vi "Lab Panel V5.25.vi"() -> ()   [LabVIEW 2017] (continued)
                    n2903 = Unbundle(w5372) -> ("CYCLE"=w5336:dbl, "MINS"=w5335:dbl, "STATUS"=w5332:string)
                    n2904 = Unbundle(w5371) -> ("CYCLE"=w5331:dbl, "MINS"=w5330:dbl, "STATUS"=w5327:string)
                    n2905 = Unbundle(w5370) -> ("CYCLE"=w5326:dbl, "MINS"=w5325:dbl, "STATUS"=w5322:string)
                    n2906 = Unbundle(w5369) -> ("CYCLE"=w5368:dbl, "MINS"=w5367:dbl, "STATUS"=w5319:string)
                    n2907 = Number To Decimal String(number=w5354) -> (decimal integer string=w5356:string)  [unwired: 1 in]
                    n2908 = Number To Decimal String(number=w5351) -> (decimal integer string=w5349:string)  [unwired: 1 in]
                    n2909 = Number To Decimal String(number=w5346) -> (decimal integer string=w5344:string)  [unwired: 1 in]
                    n2910 = Number To Decimal String(number=w5361) -> (decimal integer string=w5359:string)  [unwired: 1 in]
                    n2911 = Number To Decimal String(number=w5341) -> (decimal integer string=w5339:string)  [unwired: 1 in]
                    n2912 = Number To Decimal String(number=w5366) -> (decimal integer string=w5364:string)  [unwired: 1 in]
                    n2913 = Number To Decimal String(number=w5368) -> (decimal integer string=w5321:string)  [unwired: 1 in]
                    n2914 = Number To Decimal String(number=w5336) -> (decimal integer string=w5334:string)  [unwired: 1 in]
                    n2915 = Number To Decimal String(number=w5331) -> (decimal integer string=w5329:string)  [unwired: 1 in]
                    n2916 = Number To Decimal String(number=w5326) -> (decimal integer string=w5324:string)  [unwired: 1 in]
                    n2917 = Number To Fractional String(number=w5353, precision (6)=w5298) -> (F-format string=w5355:string)  [unwired: 2 in]
                    n2918 = Number To Fractional String(number=w5340, precision (6)=w5298) -> (F-format string=w5338:string)  [unwired: 2 in]
                    n2919 = Number To Fractional String(number=w5350, precision (6)=w5298) -> (F-format string=w5348:string)  [unwired: 2 in]
                    n2920 = Number To Fractional String(number=w5345, precision (6)=w5298) -> (F-format string=w5343:string)  [unwired: 2 in]
                    n2921 = Number To Fractional String(number=w5330, precision (6)=w5298) -> (F-format string=w5328:string)  [unwired: 2 in]
                    n2922 = Number To Fractional String(number=w5335, precision (6)=w5298) -> (F-format string=w5333:string)  [unwired: 2 in]
                    n2923 = Number To Fractional String(number=w5360, precision (6)=w5298) -> (F-format string=w5358:string)  [unwired: 2 in]
                    n2924 = Number To Fractional String(number=w5325, precision (6)=w5298) -> (F-format string=w5323:string)  [unwired: 2 in]
                    n2925 = Number To Fractional String(number=w5365, precision (6)=w5298) -> (F-format string=w5363:string)  [unwired: 2 in]
                    n2926 = Number To Fractional String(number=w5367, precision (6)=w5298) -> (F-format string=w5320:string)  [unwired: 2 in]
                    n2927 = Concatenate Strings(w5297, w5339, w5297, w5338, w5297, w5337) -> (w5313:string)
                    n2928 = Concatenate Strings(w5297, w5334, w5297, w5333, w5297, w5332) -> (w5312:string)
                    n2929 = Concatenate Strings(w5297, w5329, w5297, w5328, w5297, w5327) -> (w5311:string)
                    n2930 = Concatenate Strings(w5297, w5324, w5297, w5323, w5297, w5322) -> (w5310:string)
                    n2931 = Concatenate Strings(w5297, w5321, w5297, w5320, w5297, w5319) -> (w5309:string)
                    n2932 = Concatenate Strings(w5297, w5364, w5297, w5363, w5297, w5362) -> (w5318:string)
                    n2933 = Concatenate Strings(w5297, w5344, w5297, w5343, w5297, w5342) -> (w5314:string)
                    n2934 = Concatenate Strings(w5297, w5359, w5297, w5358, w5297, w5357) -> (w5317:string)
                    n2935 = Concatenate Strings(w5297, w5356, w5297, w5355, w5297, w5352) -> (w5316:string)
                    n2936 = Concatenate Strings(w5297, w5349, w5297, w5348, w5297, w5347) -> (w5315:string)
                    n2937 = Concatenate Strings("]", "\r") -> (w5294:string)
                    n2938 = Concatenate Strings(w5289, w5314, w5294) -> (w5304:string)
                    n2939 = Concatenate Strings(w5291, w5316, w5294) -> (w5306:string)
                    n2940 = Concatenate Strings(w5290, w5315, w5294) -> (w5305:string)
                    n2941 = Concatenate Strings(w5286, w5311, w5294) -> (w5301:string)
                    n2942 = Concatenate Strings(w5287, w5310, w5294) -> (w5302:string)
                    n2943 = Concatenate Strings(w5285, w5312, w5294) -> (w5300:string)
                    n2944 = Concatenate Strings(w5284, w5313, w5294) -> (w5299:string)
                    n2945 = Concatenate Strings(w5288, w5309, w5294) -> (w5303:string)
                    n2946 = Concatenate Strings(w5292, w5317, w5294) -> (w5307:string)
                    n2947 = Concatenate Strings(w5293, w5318, w5294) -> (w5308:string)
                    n2948 = Concatenate Strings(w5308, w5307, w5306, w5305, w5304, w5299, w5300, w5301, w5302, w5303) -> (w5277:string)
                    n2949 = Concatenate Strings("[PANEL/", "DESC/", "CYCLES/", "MINS/", "STATUS]", "\r", w5277) -> (w5276:string)
                    "MAIL REPORT" <- w5276
                    n2950 = global write "Global display 3.vi" "log all"(w5276) -> ()
                  }
                  frame #2 {
                    w5407 = "END"
                    n2951 = local read "mail control"() -> (w5408:string)
                    n2952 = case shown="False" w5403 {
                      tunnel: w5408 -> [w5432 _]
                      tunnel: w5407 -> [w5431 _]
                      tunnel: [w5430 FALSE] -> w5393
                      frame False {
                        n2953 = Equal?(x=w5432, y=w5431) -> (x = y?=w5430:bool)
                      }
                      frame True {
                      }
                    }
                    n2954 = case shown="False" w5409 {
                      tunnel: w5408 -> [w5448 _]
                      tunnel: w5407 -> [w5447 _]
                      tunnel: [w5446 FALSE] -> w5397
                      frame False {
                        n2955 = Equal?(x=w5448, y=w5447) -> (x = y?=w5446:bool)
                      }
                      frame True {
                      }
                    }
                    n2956 = case shown="False" w5406 {
                      tunnel: w5408 -> [w5444 _]
                      tunnel: w5407 -> [w5443 _]
                      tunnel: [w5442 FALSE] -> w5396
                      frame False {
                        n2957 = Equal?(x=w5444, y=w5443) -> (x = y?=w5442:bool)
                      }
                      frame True {
                      }
                    }
                    n2958 = case shown="False" w5404 {
                      tunnel: w5408 -> [w5436 _]
                      tunnel: w5407 -> [w5435 _]
                      tunnel: [w5434 FALSE] -> w5394
                      frame False {
                        n2959 = Equal?(x=w5436, y=w5435) -> (x = y?=w5434:bool)
                      }
                      frame True {
                      }
                    }
                    n2960 = case shown="False" w5405 {
                      tunnel: w5408 -> [w5440 _]
                      tunnel: w5407 -> [w5439 _]
                      tunnel: [w5438 FALSE] -> w5395
                      frame False {
                        n2961 = Equal?(x=w5440, y=w5439) -> (x = y?=w5438:bool)
                      }
                      frame True {
                      }
                    }
                    n2962 = Or(x=w5395, y=w5394) -> (x .or. y?=w5386:bool)
                    n2963 = Or(x=w5397, y=w5396) -> (x .or. y?=w5387:bool)
                    n2964 = Or(x=w5387, y=w5386) -> (x .or. y?=w5382:bool)
                    n2965 = case shown="False" w5399 {
                      tunnel: w5408 -> [w5416 _]
                      tunnel: w5407 -> [w5415 _]
                      tunnel: [w5414 FALSE] -> w5388
                      frame False {
                        n2966 = Equal?(x=w5416, y=w5415) -> (x = y?=w5414:bool)
                      }
                      frame True {
                      }
                    }
                    n2967 = case shown="False" w5398 {
                      tunnel: w5408 -> [w5412 _]
                      tunnel: w5407 -> [w5411 _]
                      tunnel: [w5410 FALSE] -> w5392
                      frame False {
                        n2968 = Equal?(x=w5412, y=w5411) -> (x = y?=w5410:bool)
                      }
                      frame True {
                      }
                    }
                    n2969 = case shown="False" w5400 {
                      tunnel: w5408 -> [w5420 _]
                      tunnel: w5407 -> [w5419 _]
                      tunnel: [w5418 FALSE] -> w5389
                      frame False {
                        n2970 = Equal?(x=w5420, y=w5419) -> (x = y?=w5418:bool)
                      }
                      frame True {
                      }
                    }
                    n2971 = case shown="False" w5402 {
                      tunnel: w5408 -> [w5428 _]
                      tunnel: w5407 -> [w5427 _]
                      tunnel: [w5426 FALSE] -> w5391
                      frame False {
                        n2972 = Equal?(x=w5428, y=w5427) -> (x = y?=w5426:bool)
                      }
                      frame True {
                      }
                    }
                    n2973 = case shown="False" w5401 {
                      tunnel: w5408 -> [w5424 _]
                      tunnel: w5407 -> [w5423 _]
                      tunnel: [w5422 FALSE] -> w5390
                      frame False {
                        n2974 = Equal?(x=w5424, y=w5423) -> (x = y?=w5422:bool)
                      }
                      frame True {
                      }
                    }
                    n2975 = Or(x=w5391, y=w5390) -> (x .or. y?=w5385:bool)
                    n2976 = Or(x=w5389, y=w5388) -> (x .or. y?=w5384:bool)
                    n2977 = Or(x=w5392, y=w5393) -> (x .or. y?=w5380:bool)
                    n2978 = Or(x=w5385, y=w5384) -> (x .or. y?=w5383:bool)
                    n2979 = Or(x=w5382, y=w5383) -> (x .or. y?=w5381:bool)
                    n2980 = Or(x=w5381, y=w5380) -> (x .or. y?=w5379:bool)
                  }
                  frame #3 {
                    n2981 = local read "on loops"() -> (w5462:dbl)
                    n2982 = local read "jig cycle"() -> (w5459:dbl)
                    n2983 = local read "Send Mail Now"() -> (w5453:bool)
                    n2984 = Add(x=w5462, y=3.0) -> (x+y=w5460:dbl)
                    n2985 = Equal?(x=w5459, y=w5460) -> (x = y?=w5454:bool)
                    n2986 = And(x=w5454, y=w5453) -> (x .and. y?=w5452:bool)
                    n2987 = And(x=w5458, y=w5454) -> (x .and. y?=w5457:bool)
                    n2988 = And(x=w5457, y=w5456) -> (x .and. y?=w5455:bool)
                    n2989 = Or(x=w5455, y=w5452) -> (x .or. y?=w5451:bool)
                    n2990 = case shown="True" w5451 {
                      tunnel: w5467 -> [_ w5473]
                      tunnel: w5466 -> [_ w5472]
                      tunnel: "Lab Panel Test Status" -> [_ w5471]
                      tunnel: w5464 -> [_ w5470]
                      tunnel: w5463 -> [_ w5469]
                      tunnel: w5450 -> [_ w5468]
                      frame False {
                      }
                      frame True {
                        n2991 = stacked-sequence {
                          tunnel: w5473 -> [w5481 _]
                          tunnel: w5472 -> [w5480 _]
                          tunnel: w5471 -> [w5479 _]
                          tunnel: w5470 -> [w5478 _]
                          tunnel: w5469 -> [w5477 _]
                          tunnel: w5468 -> [w5476 _]
                          frame #0 {
                            n2992 = call "Lab Send Mail Test.vi"("TO:"=w5481, "subject"=w5479, "from"=w5477, "out going server"=w5478, "message"=w5480) -> ("error out"=w5475:errorcluster)  [unwired: 10 in]
                            n2993 = Bundle(cluster=w5476, "mail error"=w5475) -> (w5474:T7)  [unwired: 6 in]
                            n2994 = local write "MAIL SETTINGS"(w5474) -> ()
                          }
                          frame #1 {
                            n2995 = local write "mail control"("") -> ()
                            n2996 = local write "Send Mail Now"(FALSE) -> ()
                          }
                        }
                      }
                    }
                  }
                }
              }
            }
          }
          frame #19 {
            # "save jig cycle values once all run switches are off"
            n2997 = stacked-sequence {
              tunnel: w5493 -> [_ w5522]
              tunnel: w5492 -> [_ w5521]
              tunnel: w5491 -> [_ w5520]
              tunnel: w5490 -> [_ w5519]
              tunnel: w5489 -> [_ w5518]
              tunnel: w5488 -> [_ w5517]
              tunnel: w5487 -> [_ w5516]
              tunnel: w5486 -> [_ w5515]
              tunnel: w5485 -> [_ w5514]
              tunnel: w5484 -> [_ w5513]
              frame #0 {
              }
              frame #1 {
                n2998 = Not(x=w5513) -> (.not. x?=w5496:bool)
                n2999 = Not(x=w5521) -> (.not. x?=w5511:bool)
                n3000 = Not(x=w5518) -> (.not. x?=w5506:bool)
                n3001 = Not(x=w5516) -> (.not. x?=w5502:bool)
                n3002 = Not(x=w5514) -> (.not. x?=w5498:bool)
                n3003 = Not(x=w5522) -> (.not. x?=w5512:bool)
                n3004 = Not(x=w5520) -> (.not. x?=w5510:bool)
                n3005 = Not(x=w5517) -> (.not. x?=w5504:bool)
                n3006 = Not(x=w5519) -> (.not. x?=w5508:bool)
                n3007 = Not(x=w5515) -> (.not. x?=w5500:bool)
                n3008 = local read "Save JC"() -> (w5524:bool)
                n3009 = And(x=w5512, y=w5511) -> (x .and. y?=w5509:bool)
                n3010 = And(x=w5509, y=w5510) -> (x .and. y?=w5507:bool)
                n3011 = And(x=w5507, y=w5508) -> (x .and. y?=w5505:bool)
                n3012 = And(x=w5505, y=w5506) -> (x .and. y?=w5503:bool)
                n3013 = And(x=w5503, y=w5504) -> (x .and. y?=w5501:bool)
                n3014 = And(x=w5501, y=w5502) -> (x .and. y?=w5499:bool)
                n3015 = And(x=w5499, y=w5500) -> (x .and. y?=w5497:bool)
                n3016 = And(x=w5497, y=w5498) -> (x .and. y?=w5495:bool)
                n3017 = And(x=w5495, y=w5496) -> (x .and. y?=w5494:bool)
                n3018 = And(x=w5494, y=w5524) -> (x .and. y?=w5523:bool)
                n3019 = case shown="True" w5523 {
                  tunnel: w5494 -> [w5525 _]
                  frame False {
                    n3020 = case shown="False" w5525 {
                      frame False {
                        n3021 = local write "Save JC"(TRUE) -> ()
                      }
                      frame True {
                      }
                    }
                  }
                  frame True {
                    n3022 = stacked-sequence {
                      frame #0 {
                        n3023 = String To Path(string="c:\\crabtree\\Jig Cycles\\") -> (path=w5537:path)
                        n3024 = Build Path(base path=w5537, name or relative path="jigcycles.bin") -> (appended path=w5535:path)
                        n3025 = Create Folder(path (use dialog)=w5537) -> (error out=w5539:errorcluster)  [unwired: 2 in, 2 out]
                        n3026 = local read "JIG RELAY CYCLES"() -> (w5529:T8)
                        n3027 = call <vilib>:"Clear Errors.vi"("error in (no error)"=w5539) -> ()  [unwired: 5 in, 2 out]
                        n3028 = local write "Save JC"(FALSE) -> ()
                        n3029 = Open/Create/Replace File(file path (use dialog)=w5535, operation (0:open)=T17."replace or create") -> (refnum out=w5533:refnum<file>, error out=w5534:errorcluster)  [unwired: 4 in, 1 out]
                        n3030 = Write to Binary File(file (use dialog)=w5533, data=w5529, error in=w5534) -> (refnum out=w5532:refnum<file>, error out=w5531:errorcluster)  [unwired: 3 in, 1 out]
                        n3031 = Close File(refnum=w5532, error in=w5531) -> (error out=w5530:errorcluster)  [unwired: 1 out]
                        n3032 = local write "data file error"(w5530) -> ()
                      }
                      frame #1 {
                        n3033 = local read "JIG RELAY CYCLES"() -> (w5562:T8)
                        n3034 = Unbundle By Name(w5562) -> ("LAB01-1"=w5557:dbl, "LAB01-2"=w5556:dbl, "LAB02-1"=w5554:dbl, "LAB02-2"=w5553:dbl, "LAB03-1"=w5551:dbl, "LAB03-2"=w5548:dbl, "LAB04-1"=w5547:dbl, "LAB04-2"=w5545:dbl, "LAB05-1"=w5543:dbl, "LAB05-2"=w5541:dbl)
                        n3035 = stacked-sequence {
                          tunnel: w5557 -> [w5565 _ _ _ _ _ _ _ _ _]
                          tunnel: 1000000 -> [w5568 w5578 w5588 w5598 w5608 w5618 w5628 w5638 w5648 w5658]
                          tunnel: [w5566 _ _ _ _ _ _ _ _ _] -> w5560
                          tunnel: "TEST STATION HAS REACHED 1 MILLION CYCLES, REPLACE  CONTROL RELAYS" -> [w5564 w5576 w5586 w5596 w5606 w5616 w5626 w5636 w5646 w5656]
                          tunnel: [_ w5575 _ _ _ _ _ _ _ _] -> w5558
                          tunnel: w5556 -> [_ w5574 _ _ _ _ _ _ _ _]
                          tunnel: [_ _ w5585 _ _ _ _ _ _ _] -> w5555
                          tunnel: w5554 -> [_ _ w5584 _ _ _ _ _ _ _]
                          tunnel: w5553 -> [_ _ _ w5595 _ _ _ _ _ _]
                          tunnel: [_ _ _ w5594 _ _ _ _ _ _] -> w5552
                          tunnel: w5551 -> [_ _ _ _ w5605 _ _ _ _ _]
                          tunnel: [_ _ _ _ w5604 _ _ _ _ _] -> w5550
                          tunnel: [_ _ _ _ _ w5615 _ _ _ _] -> w5549
                          tunnel: w5548 -> [_ _ _ _ _ w5614 _ _ _ _]
                          tunnel: w5547 -> [_ _ _ _ _ _ w5625 _ _ _]
                          tunnel: [_ _ _ _ _ _ w5624 _ _ _] -> w5546
                          tunnel: w5545 -> [_ _ _ _ _ _ _ w5635 _ _]
                          tunnel: [_ _ _ _ _ _ _ w5634 _ _] -> w5544
                          tunnel: w5543 -> [_ _ _ _ _ _ _ _ w5645 _]
                          tunnel: [_ _ _ _ _ _ _ _ w5644 _] -> w5542
                          tunnel: w5541 -> [_ _ _ _ _ _ _ _ _ w5655]
                          tunnel: [_ _ _ _ _ _ _ _ _ w5654] -> w5540
                          frame #0 {
                            n3036 = Greater?(x=w5565, y=w5568) -> (0:w5567:bool)
                            n3037 = case shown="True" w5567 {
                              tunnel: [w5569 0] -> w5566
                              tunnel: w5565 -> [w5569 _]
                              tunnel: w5564 -> [_ w5570]
                              frame False {
                              }
                              frame True {
                                n3038 = Concatenate Strings("LA01-1 ", w5570) -> (w5573:string)
                                n3039 = One Button Dialog(message=w5573) -> ()  [unwired: 1 in, 1 out]
                              }
                            }
                          }
                          frame #1 {
                            n3040 = Greater?(x=w5574, y=w5578) -> (0:w5577:bool)
                            n3041 = case shown="True" w5577 {
                              tunnel: [w5579 0] -> w5575
                              tunnel: w5574 -> [w5579 _]
                              tunnel: w5576 -> [_ w5580]
                              frame False {
                              }
                              frame True {
                                n3042 = Concatenate Strings("LA01-2 ", w5580) -> (w5583:string)
                                n3043 = One Button Dialog(message=w5583) -> ()  [unwired: 1 in, 1 out]
                              }
                            }
                          }
                          frame #2 {
                            n3044 = Greater?(x=w5584, y=w5588) -> (0:w5587:bool)
                            n3045 = case shown="True" w5587 {
                              tunnel: [w5589 0] -> w5585
                              tunnel: w5584 -> [w5589 _]
                              tunnel: w5586 -> [_ w5590]
                              frame False {
                              }
                              frame True {
                                n3046 = Concatenate Strings("LA02-1 ", w5590) -> (w5593:string)
                                n3047 = One Button Dialog(message=w5593) -> ()  [unwired: 1 in, 1 out]
                              }
                            }
                          }
                          frame #3 {
                            n3048 = Greater?(x=w5595, y=w5598) -> (0:w5597:bool)
                            n3049 = case shown="True" w5597 {
                              tunnel: [w5599 0] -> w5594
                              tunnel: w5595 -> [w5599 _]
                              tunnel: w5596 -> [_ w5600]
                              frame False {
                              }
                              frame True {
                                n3050 = Concatenate Strings("LA02-2 ", w5600) -> (w5603:string)
                                n3051 = One Button Dialog(message=w5603) -> ()  [unwired: 1 in, 1 out]
                              }
                            }
                          }
                          frame #4 {
                            n3052 = Greater?(x=w5605, y=w5608) -> (0:w5607:bool)
                            n3053 = case shown="True" w5607 {
                              tunnel: [w5609 0] -> w5604
                              tunnel: w5605 -> [w5609 _]
                              tunnel: w5606 -> [_ w5610]
                              frame False {
                              }
                              frame True {
                                n3054 = Concatenate Strings("LA03-1 ", w5610) -> (w5613:string)
                                n3055 = One Button Dialog(message=w5613) -> ()  [unwired: 1 in, 1 out]
                              }
                            }
                          }
                          frame #5 {
                            n3056 = Greater?(x=w5614, y=w5618) -> (0:w5617:bool)
                            n3057 = case shown="True" w5617 {
                              tunnel: [w5619 0] -> w5615
                              tunnel: w5614 -> [w5619 _]
                              tunnel: w5616 -> [_ w5620]
                              frame False {
                              }
                              frame True {
                                n3058 = Concatenate Strings("LA03-2 ", w5620) -> (w5623:string)
                                n3059 = One Button Dialog(message=w5623) -> ()  [unwired: 1 in, 1 out]
                              }
                            }
                          }
                          frame #6 {
                            n3060 = Greater?(x=w5625, y=w5628) -> (0:w5627:bool)
                            n3061 = case shown="True" w5627 {
                              tunnel: [w5629 0] -> w5624
                              tunnel: w5625 -> [w5629 _]
                              tunnel: w5626 -> [_ w5630]
                              frame False {
                              }
                              frame True {
                                n3062 = Concatenate Strings("LA04-1 ", w5630) -> (w5633:string)
                                n3063 = One Button Dialog(message=w5633) -> ()  [unwired: 1 in, 1 out]
                              }
                            }
                          }
                          frame #7 {
                            n3064 = Greater?(x=w5635, y=w5638) -> (0:w5637:bool)
                            n3065 = case shown="True" w5637 {
                              tunnel: [w5639 0] -> w5634
                              tunnel: w5635 -> [w5639 _]
                              tunnel: w5636 -> [_ w5640]
                              frame False {
                              }
                              frame True {
                                n3066 = Concatenate Strings("LA04-2 ", w5640) -> (w5643:string)
                                n3067 = One Button Dialog(message=w5643) -> ()  [unwired: 1 in, 1 out]
                              }
                            }
                          }
                          frame #8 {
                            n3068 = Greater?(x=w5645, y=w5648) -> (0:w5647:bool)
                            n3069 = case shown="True" w5647 {
                              tunnel: [w5649 0] -> w5644
                              tunnel: w5645 -> [w5649 _]
                              tunnel: w5646 -> [_ w5650]
                              frame False {
                              }
                              frame True {
                                n3070 = Concatenate Strings("LA05-1 ", w5650) -> (w5653:string)
                                n3071 = One Button Dialog(message=w5653) -> ()  [unwired: 1 in, 1 out]
                              }
                            }
                          }
                          frame #9 {
                            n3072 = Greater?(x=w5655, y=w5658) -> (0:w5657:bool)
                            n3073 = case shown="True" w5657 {
                              tunnel: [w5659 0] -> w5654
                              tunnel: w5655 -> [w5659 _]
                              tunnel: w5656 -> [_ w5660]
                              frame False {
                              }
                              frame True {
                                n3074 = Concatenate Strings("LA05-2 ", w5660) -> (w5663:string)
                                n3075 = One Button Dialog(message=w5663) -> ()  [unwired: 1 in, 1 out]
                              }
                            }
                          }
                        }
                        n3076 = Bundle By Name(cluster=w5562, "LAB01-1"=w5560, "LAB01-2"=w5558, "LAB02-1"=w5555, "LAB02-2"=w5552, "LAB03-1"=w5550, "LAB03-2"=w5549, "LAB04-1"=w5546, "LAB04-2"=w5544, "LAB05-1"=w5542, "LAB05-2"=w5540) -> (w5561:T8)
                        n3077 = local write "JIG RELAY CYCLES"(w5561) -> ()
                      }
                    }
                  }
                }
              }
            }
          }
          frame #20 {
            # "get temperature values"
            n3078 = local read "Simulate"() -> (w5676:bool)
            n3079 = local read "Temp Test Cal"() -> (w5673:dbl)
            n3080 = stacked-sequence {
              seq-local: [w5678 _] -> [_ w5723]
              tunnel: w5676 -> [_ w5736]
              tunnel: T14 {"1  (A) cal"=1.0, "1 (V) cal"=1.0, "1 (PF) cal"=1.0, "1 (TL) cal"=1.0, "1 (TN) cal"=1.0, "2 (A) cal"=1.0, "2 (V) cal"=1.0, "2 (PF) cal"=1.0, "2 (TL) cal"=1.0, "2 (TN) cal"=1.0} ("CAL LAB01") -> [_ w5735]
              tunnel: w5674 -> [_ w5734]
              tunnel: w5673 -> [_ w5733]
              tunnel: w5672 -> [_ w5732]
              tunnel: w5671 -> [_ w5731]
              tunnel: w5670 -> [_ w5730]
              tunnel: w5669 -> [_ w5729]
              tunnel: w5668 -> [_ w5728]
              tunnel: w5667 -> [_ w5727]
              tunnel: w5666 -> [_ w5726]
              tunnel: w5665 -> [_ w5725]
              tunnel: w5664 -> [_ w5724]
              frame #0 {
                # "only get temperature from initial valid temperature circuits"
                n3081 = local read "Select COM port"() -> (w5686:refnum<visa-resource-name>)
                "COM port" <- w5686
                n3082 = global write "Global 1.vi" "COM port"(w5686) -> ()
                n3083 = global write "Global 1.vi" "tmp dly lps"("Temp Delay Lps") -> ()
                n3084 = local read "Temp read loop"() -> (w5683:dbl)
                n3085 = global write "Global 1.vi" "dly value"("Temp Value") -> ()
                n3086 = local read "jig cycle"() -> (w5687:dbl)
                n3087 = local read "on loops"() -> (w5689:dbl)
                n3088 = Equal?(x=w5683, y=1) -> (x = y?=w5680:bool)
                n3089 = Add(x=w5689, y=3) -> (x+y=w5690:dbl)
                n3090 = Equal?(x=w5687, y=w5690) -> (x = y?=w5681:bool)
                n3091 = And(x=w5681, y=w5680) -> (x .and. y?=w5679:bool)
                n3092 = Or(x=w5679, y="Read Temp") -> (x .or. y?=w5678:bool)
                n3093 = case shown="True" w5678 {
                  frame False {
                  }
                  frame True {
                    n3094 = local read "Simulate"() -> (w5692:bool)
                    n3095 = local write "TEMP"(TRUE) -> ()
                    n3096 = local write "Read Temp"(FALSE) -> ()
                    n3097 = stacked-sequence {
                      tunnel: 1.0 -> [_ _ _ _ w5722]
                      tunnel: w5692 -> [_ _ _ _ w5721]
                      frame #0 {
                        # "only switch relay on to reset temp circuits if busy testing"
                        n3098 = disable-structure shown="Disabled" {
                          frame Disabled {
                            n3099 = local read "Any Test Running"() -> ()  [unwired: 1 out]
                          }
                          frame Enabled {
                          }
                        }
                        n3100 = local read "USB OUT 0"() -> (w5696:bool[])
                        n3101 = local read "USB OUT 2"() -> (w5698:bool[])
                        n3102 = local read "USB OUT 1"() -> (w5697:bool[])
                        n3103 = Insert Into Array(array=w5698, index=7, new element=TRUE) -> (w5699:bool[])
                        n3104 = call "sub vi - Drive Relays All v6.vi"("Array #2"=w5699, "Array #1"=w5697, "Array #0"=w5696) -> ()  [unwired: 8 in, 1 out]
                      }
                      frame #1 {
                        # "time delay"
                        n3105 = Wait (ms)(milliseconds to wait=500) -> ()  [unwired: 1 out]
                      }
                      frame #2 {
                        # "switch relay off"
                        n3106 = local read "USB OUT 0"() -> (w5702:bool[])
                        n3107 = local read "USB OUT 2"() -> (w5704:bool[])
                        n3108 = local read "USB OUT 1"() -> (w5703:bool[])
                        n3109 = Insert Into Array(array=w5704, index=7, new element=FALSE) -> (w5705:bool[])
                        n3110 = call "sub vi - Drive Relays All v6.vi"("Array #2"=w5705, "Array #1"=w5703, "Array #0"=w5702) -> ()  [unwired: 8 in, 1 out]
                      }
                      frame #3 {
                        # "time delay"
                        n3111 = Wait (ms)(milliseconds to wait=200) -> ()  [unwired: 1 out]
                      }
                      frame #4 {
                        # "read all valid temp circuits"
                        n3112 = local read "LAB01-TP"() -> (w5714:bool)
                        n3113 = local read "LAB03-TP"() -> (w5712:bool)
                        n3114 = local read "LAB02-TP"() -> (w5713:bool)
                        n3115 = local read "LAB04-TP"() -> (w5711:bool)
                        n3116 = local read "LAB05-TP"() -> (w5715:bool)
                        n3117 = call "sub vi - GET ALL TEMP v7.vi"("LA01-EN"=w5714, "simulate"=w5721, "LA02-EN"=w5713, "LA03-EN"=w5712, "LA04-EN"=w5711, "LA05-EN"=w5715, "Gen Cal Value"=w5722) -> ("LOOP TIME"=→"Read Time":dbl, "LA01 TEMP"=w5720:T25, "LA02 TEMP"=w5719:T25, "LA03 TEMP"=w5718:T25, "LA04 TEMP"=w5717:T25, "error"=→"Error Temp":bool, "LA05 TEMP"=w5716:T25)  [unwired: 1 in, 1 out]
                        n3118 = local write "LAB01 TEMP"(w5720) -> ()
                        n3119 = local write "LAB02 TEMP"(w5719) -> ()
                        n3120 = local write "LAB03 TEMP"(w5718) -> ()
                        n3121 = local write "LAB04 TEMP"(w5717) -> ()
                        n3122 = local write "LAB05 TEMP"(w5716) -> ()
                      }
                    }
                  }
                }
              }
              frame #1 {
                n3123 = case shown="True" w5723 {
                  tunnel: w5736 -> [_ w5749]
                  tunnel: w5735 -> [_ w5748]
                  tunnel: w5734 -> [_ w5747]
                  tunnel: w5733 -> [_ w5746]
                  tunnel: w5732 -> [_ w5745]
                  tunnel: w5731 -> [_ w5744]
                  tunnel: w5730 -> [_ w5743]
                  tunnel: w5729 -> [_ w5742]
                  tunnel: w5728 -> [_ w5741]
                  tunnel: w5727 -> [_ w5740]
                  tunnel: w5726 -> [_ w5739]
                  tunnel: w5725 -> [_ w5738]
                  tunnel: w5724 -> [_ w5737]
                  frame False {
                  }
                  frame True {
                    n3124 = stacked-sequence {
                      tunnel: w5749 -> [_ w5762 w5807 w5852 w5897 w5942]
                      tunnel: w5748 -> [_ w5761 w5806 w5851 w5896 w5941]
                      tunnel: w5747 -> [_ w5751 _ _ _ _]
                      tunnel: w5746 -> [_ w5756 w5805 w5850 w5895 w5940]
                      tunnel: w5745 -> [_ w5750 _ _ _ _]
                      tunnel: w5744 -> [_ _ w5796 _ _ _]
                      tunnel: w5743 -> [_ _ w5795 _ _ _]
                      tunnel: w5742 -> [_ _ _ w5841 _ _]
                      tunnel: w5741 -> [_ _ _ w5840 _ _]
                      tunnel: w5740 -> [_ _ _ _ w5886 _]
                      tunnel: w5739 -> [_ _ _ _ w5885 _]
                      tunnel: w5738 -> [_ _ _ _ _ w5931]
                      tunnel: w5737 -> [_ _ _ _ _ w5930]
                      frame #0 {
                      }
                      frame #1 {
                        n3125 = case shown="False" w5762 {
                          tunnel: [w5793 w5794] -> w5778
                          tunnel: w5761 -> [_ w5794]
                          frame False {
                            n3126 = local read "CAL LAB01"() -> (w5793:T14)
                          }
                          frame True {
                          }
                        }
                        n3127 = local read "TEMP LA01"() -> (w5769:T9)
                        n3128 = local read "LAB01 TEMP"() -> (w5768:T12)
                        n3129 = call "sub vi - temperature delay v3.vi"("2-run"=w5750, "1-run"=w5751, "temp values IN"=w5769, "temp signals"=w5768) -> ("T2-N"=w5764:dbl, "T2-L"=w5765:dbl, "T1-N"=w5766:dbl, "T1-L"=w5767:dbl, "temp values OUT"=w5763:T44)  [unwired: 3 in]
                        n3130 = Unbundle By Name(w5778) -> ("1 (TL) cal"=w5773:dbl, "1 (TN) cal"=w5772:dbl, "2 (TL) cal"=w5771:dbl, "2 (TN) cal"=w5770:dbl)  [unwired: 6 out]
                        n3131 = local write "TEMP LA01"(w5763) -> ()
                        n3132 = Multiply(x=w5767, y=w5773) -> (x*y=w5760:dbl)
                        n3133 = Multiply(x=w5766, y=w5772) -> (x*y=w5758:dbl)
                        n3134 = Multiply(x=w5765, y=w5771) -> (x*y=w5755:dbl)
                        n3135 = Multiply(x=w5764, y=w5770) -> (x*y=w5754:dbl)
                        n3136 = case shown="True" w5751 {
                          tunnel: w5760 -> [w5787 w5792]
                          tunnel: w5756 -> [_ w5790]
                          tunnel: [w5787 w5791] -> w5759
                          tunnel: w5758 -> [w5786 w5789]
                          tunnel: [w5786 w5788] -> w5757
                          frame False {
                          }
                          frame True {
                            n3137 = Multiply(x=w5790, y=w5789) -> (x*y=w5788:dbl)
                            n3138 = Multiply(x=w5790, y=w5792) -> (x*y=w5791:dbl)
                          }
                        }
                        n3139 = case shown="True" w5750 {
                          tunnel: w5755 -> [w5780 w5785]
                          tunnel: w5756 -> [_ w5783]
                          tunnel: [w5780 w5784] -> w5753
                          tunnel: w5754 -> [w5779 w5782]
                          tunnel: [w5779 w5781] -> w5752
                          frame False {
                          }
                          frame True {
                            n3140 = Multiply(x=w5783, y=w5782) -> (x*y=w5781:dbl)
                            n3141 = Multiply(x=w5783, y=w5785) -> (x*y=w5784:dbl)
                          }
                        }
                        n3142 = local read "SIG LAB01-2"() -> (w5775:T2)
                        n3143 = local read "SIG LAB01-1"() -> (w5777:T2)
                        n3144 = Bundle By Name(cluster=w5777, "Tmp Live"=w5759, "Tmp Neut"=w5757) -> (w5776:T2)
                        n3145 = Bundle By Name(cluster=w5775, "Tmp Live"=w5753, "Tmp Neut"=w5752) -> (w5774:T2)
                        n3146 = local write "SIG LAB01-1"(w5776) -> ()
                        n3147 = local write "SIG LAB01-2"(w5774) -> ()
                      }
                      frame #2 {
                        n3148 = case shown="True" w5807 {
                          tunnel: [w5838 w5839] -> w5823
                          tunnel: w5806 -> [_ w5839]
                          frame False {
                            n3149 = local read "CAL LAB02"() -> (w5838:T15)
                          }
                          frame True {
                          }
                        }
                        n3150 = local read "LAB02 TEMP"() -> (w5814:T12)
                        n3151 = local read "TEMP LA02"() -> (w5813:T9)
                        n3152 = call "sub vi - temperature delay v3.vi"("2-run"=w5795, "1-run"=w5796, "temp values IN"=w5813, "temp signals"=w5814) -> ("T2-N"=w5808:dbl, "T2-L"=w5809:dbl, "T1-N"=w5810:dbl, "T1-L"=w5811:dbl, "temp values OUT"=w5812:T44)  [unwired: 3 in]
                        n3153 = Unbundle By Name(w5823) -> ("1 (TL) cal"=w5818:dbl, "1 (TN) cal"=w5817:dbl, "2 (TL) cal"=w5816:dbl, "2 (TN) cal"=w5815:dbl)  [unwired: 6 out]
                        n3154 = local write "TEMP LA02"(w5812) -> ()
                        n3155 = Multiply(x=w5811, y=w5818) -> (x*y=w5804:dbl)
                        n3156 = Multiply(x=w5810, y=w5817) -> (x*y=w5803:dbl)
                        n3157 = Multiply(x=w5809, y=w5816) -> (x*y=w5800:dbl)
                        n3158 = Multiply(x=w5808, y=w5815) -> (x*y=w5799:dbl)
                        n3159 = case shown="True" w5796 {
                          tunnel: w5804 -> [w5832 w5837]
                          tunnel: w5805 -> [_ w5835]
                          tunnel: [w5832 w5836] -> w5802
                          tunnel: w5803 -> [w5831 w5834]
                          tunnel: [w5831 w5833] -> w5801
                          frame False {
                          }
                          frame True {
                            n3160 = Multiply(x=w5835, y=w5834) -> (x*y=w5833:dbl)
                            n3161 = Multiply(x=w5835, y=w5837) -> (x*y=w5836:dbl)
                          }
                        }
                        n3162 = case shown="True" w5795 {
                          tunnel: w5800 -> [w5825 w5830]
                          tunnel: w5805 -> [_ w5828]
                          tunnel: [w5825 w5829] -> w5798
                          tunnel: w5799 -> [w5824 w5827]
                          tunnel: [w5824 w5826] -> w5797
                          frame False {
                          }
                          frame True {
                            n3163 = Multiply(x=w5828, y=w5827) -> (x*y=w5826:dbl)
                            n3164 = Multiply(x=w5828, y=w5830) -> (x*y=w5829:dbl)
                          }
                        }
                        n3165 = local read "SIG LAB02-2"() -> (w5820:T2)
                        n3166 = local read "SIG LAB02-1"() -> (w5822:T2)
                        n3167 = Bundle By Name(cluster=w5822, "Tmp Live"=w5802, "Tmp Neut"=w5801) -> (w5821:T2)
                        n3168 = Bundle By Name(cluster=w5820, "Tmp Live"=w5798, "Tmp Neut"=w5797) -> (w5819:T2)
                        n3169 = local write "SIG LAB02-1"(w5821) -> ()
                        n3170 = local write "SIG LAB02-2"(w5819) -> ()
                      }
                      frame #3 {
                        n3171 = case shown="False" w5852 {
                          tunnel: [w5883 w5884] -> w5868
                          tunnel: w5851 -> [_ w5884]
                          frame False {
                            n3172 = local read "CAL LAB03"() -> (w5883:T14)
                          }
                          frame True {
                          }
                        }
                        n3173 = local read "TEMP LA03"() -> (w5858:T9)
                        n3174 = local read "LAB03 TEMP"() -> (w5859:T12)
                        n3175 = call "sub vi - temperature delay v3.vi"("2-run"=w5840, "1-run"=w5841, "temp values IN"=w5858, "temp signals"=w5859) -> ("T2-N"=w5853:dbl, "T2-L"=w5854:dbl, "T1-N"=w5855:dbl, "T1-L"=w5856:dbl, "temp values OUT"=w5857:T44)  [unwired: 3 in]
                        n3176 = Unbundle By Name(w5868) -> ("1 (TL) cal"=w5863:dbl, "1 (TN) cal"=w5862:dbl, "2 (TL) cal"=w5861:dbl, "2 (TN) cal"=w5860:dbl)  [unwired: 6 out]
                        n3177 = local write "TEMP LA03"(w5857) -> ()
                        n3178 = Multiply(x=w5856, y=w5863) -> (x*y=w5849:dbl)
                        n3179 = Multiply(x=w5855, y=w5862) -> (x*y=w5848:dbl)
                        n3180 = Multiply(x=w5854, y=w5861) -> (x*y=w5845:dbl)
                        n3181 = Multiply(x=w5853, y=w5860) -> (x*y=w5844:dbl)
                        n3182 = case shown="True" w5840 {
                          tunnel: w5845 -> [w5870 w5875]
                          tunnel: w5850 -> [_ w5873]
                          tunnel: [w5870 w5874] -> w5843
                          tunnel: w5844 -> [w5869 w5872]
                          tunnel: [w5869 w5871] -> w5842
                          frame False {
                          }
                          frame True {
                            n3183 = Multiply(x=w5873, y=w5872) -> (x*y=w5871:dbl)
                            n3184 = Multiply(x=w5873, y=w5875) -> (x*y=w5874:dbl)
                          }
                        }
                        n3185 = case shown="True" w5841 {
                          tunnel: w5849 -> [w5877 w5882]
                          tunnel: w5850 -> [_ w5880]
                          tunnel: [w5877 w5881] -> w5847
                          tunnel: w5848 -> [w5876 w5879]
                          tunnel: [w5876 w5878] -> w5846
                          frame False {
                          }
                          frame True {
                            n3186 = Multiply(x=w5880, y=w5879) -> (x*y=w5878:dbl)
                            n3187 = Multiply(x=w5880, y=w5882) -> (x*y=w5881:dbl)
                          }
                        }
                        n3188 = local read "SIG LAB03-2"() -> (w5865:T2)
                        n3189 = local read "SIG LAB03-1"() -> (w5867:T2)
                        n3190 = Bundle By Name(cluster=w5867, "Tmp Live"=w5847, "Tmp Neut"=w5846) -> (w5866:T2)
                        n3191 = Bundle By Name(cluster=w5865, "Tmp Live"=w5843, "Tmp Neut"=w5842) -> (w5864:T2)
                        n3192 = local write "SIG LAB03-1"(w5866) -> ()
                        n3193 = local write "SIG LAB03-2"(w5864) -> ()
                      }
                      frame #4 {
                        n3194 = case shown="False" w5897 {
                          tunnel: [w5928 w5929] -> w5913
                          tunnel: w5896 -> [_ w5929]
                          frame False {
                            n3195 = local read "CAL LAB04"() -> (w5928:T14)
                          }
                          frame True {
                          }
                        }
                        n3196 = local read "LAB04 TEMP"() -> (w5903:T12)
                        n3197 = local read "TEMP LA04"() -> (w5904:T9)
                        n3198 = call "sub vi - temperature delay v3.vi"("2-run"=w5885, "1-run"=w5886, "temp values IN"=w5904, "temp signals"=w5903) -> ("T2-N"=w5898:dbl, "T2-L"=w5899:dbl, "T1-N"=w5900:dbl, "T1-L"=w5901:dbl, "temp values OUT"=w5902:T44)  [unwired: 3 in]
                        n3199 = Unbundle By Name(w5913) -> ("1 (TL) cal"=w5908:dbl, "1 (TN) cal"=w5907:dbl, "2 (TL) cal"=w5906:dbl, "2 (TN) cal"=w5905:dbl)  [unwired: 6 out]
                        n3200 = local write "TEMP LA04"(w5902) -> ()
                        n3201 = Multiply(x=w5901, y=w5908) -> (x*y=w5894:dbl)
                        n3202 = Multiply(x=w5900, y=w5907) -> (x*y=w5893:dbl)
                        n3203 = Multiply(x=w5899, y=w5906) -> (x*y=w5890:dbl)
                        n3204 = Multiply(x=w5898, y=w5905) -> (x*y=w5889:dbl)
                        n3205 = case shown="True" w5885 {
                          tunnel: w5890 -> [w5915 w5920]
                          tunnel: w5895 -> [_ w5918]
                          tunnel: [w5915 w5919] -> w5888
                          tunnel: w5889 -> [w5914 w5917]
                          tunnel: [w5914 w5916] -> w5887
                          frame False {
                          }
                          frame True {
                            n3206 = Multiply(x=w5918, y=w5917) -> (x*y=w5916:dbl)
                            n3207 = Multiply(x=w5918, y=w5920) -> (x*y=w5919:dbl)
                          }
                        }
                        n3208 = case shown="True" w5886 {
                          tunnel: w5894 -> [w5922 w5927]
                          tunnel: w5895 -> [_ w5925]
                          tunnel: [w5922 w5926] -> w5892
                          tunnel: w5893 -> [w5921 w5924]
                          tunnel: [w5921 w5923] -> w5891
                          frame False {
                          }
                          frame True {
                            n3209 = Multiply(x=w5925, y=w5924) -> (x*y=w5923:dbl)
                            n3210 = Multiply(x=w5925, y=w5927) -> (x*y=w5926:dbl)
                          }
                        }
                        n3211 = local read "SIG LAB04-2"() -> (w5910:T2)
                        n3212 = local read "SIG LAB04-1"() -> (w5912:T2)
                        n3213 = Bundle By Name(cluster=w5912, "Tmp Live"=w5892, "Tmp Neut"=w5891) -> (w5911:T2)
                        n3214 = Bundle By Name(cluster=w5910, "Tmp Live"=w5888, "Tmp Neut"=w5887) -> (w5909:T2)
                        n3215 = local write "SIG LAB04-1"(w5911) -> ()
                        n3216 = local write "SIG LAB04-2"(w5909) -> ()
                      }
                      frame #5 {
                        n3217 = case shown="False" w5942 {
                          tunnel: [w5973 w5974] -> w5958
                          tunnel: w5941 -> [_ w5974]
                          frame False {
                            n3218 = local read "CAL LAB05"() -> (w5973:T14)
                          }
                          frame True {
                          }
                        }
                        n3219 = local read "LAB05 TEMP"() -> (w5948:T12)
                        n3220 = local read "TEMP LA05"() -> (w5949:T9)
                        n3221 = call "sub vi - temperature delay v3.vi"("2-run"=w5930, "1-run"=w5931, "temp values IN"=w5949, "temp signals"=w5948) -> ("T2-N"=w5944:dbl, "T2-L"=w5945:dbl, "T1-N"=w5946:dbl, "T1-L"=w5947:dbl, "temp values OUT"=w5943:T44)  [unwired: 3 in]
                        n3222 = local write "TEMP LA05"(w5943) -> ()
                        n3223 = Unbundle By Name(w5958) -> ("1 (TL) cal"=w5950:dbl, "1 (TN) cal"=w5953:dbl, "2 (TL) cal"=w5952:dbl, "2 (TN) cal"=w5951:dbl)  [unwired: 6 out]
                        n3224 = Multiply(x=w5947, y=w5950) -> (x*y=w5939:dbl)
                        n3225 = Multiply(x=w5946, y=w5953) -> (x*y=w5938:dbl)
                        n3226 = Multiply(x=w5945, y=w5952) -> (x*y=w5935:dbl)
                        n3227 = Multiply(x=w5944, y=w5951) -> (x*y=w5934:dbl)
                        n3228 = case shown="True" w5930 {
                          tunnel: w5935 -> [w5960 w5965]
                          tunnel: w5940 -> [_ w5963]
                          tunnel: [w5960 w5964] -> w5933
                          tunnel: w5934 -> [w5959 w5962]
                          tunnel: [w5959 w5961] -> w5932
                          frame False {
                          }
                          frame True {
                            n3229 = Multiply(x=w5963, y=w5962) -> (x*y=w5961:dbl)
                            n3230 = Multiply(x=w5963, y=w5965) -> (x*y=w5964:dbl)
                          }
                        }
                        n3231 = case shown="True" w5931 {
                          tunnel: w5939 -> [w5967 w5972]
                          tunnel: w5940 -> [_ w5970]
                          tunnel: [w5967 w5971] -> w5937
                          tunnel: w5938 -> [w5966 w5969]
                          tunnel: [w5966 w5968] -> w5936
                          frame False {
                          }
                          frame True {
                            n3232 = Multiply(x=w5970, y=w5969) -> (x*y=w5968:dbl)
